vi "Find Default Node Details.vi"(6 "Node Type":string(combo)="DefaultChannelNodes", 8 "error in":errorcluster, 11 "Section Node":refnum<k20>) -> (0 "error out":errorcluster, 3 "Default Node Details":cluster{"Name":string, "TypeName":string}[](array[cluster]))   [LabVIEW 2025]
uses:
  <resource>/objmgr/DOMUserDefRef.rc
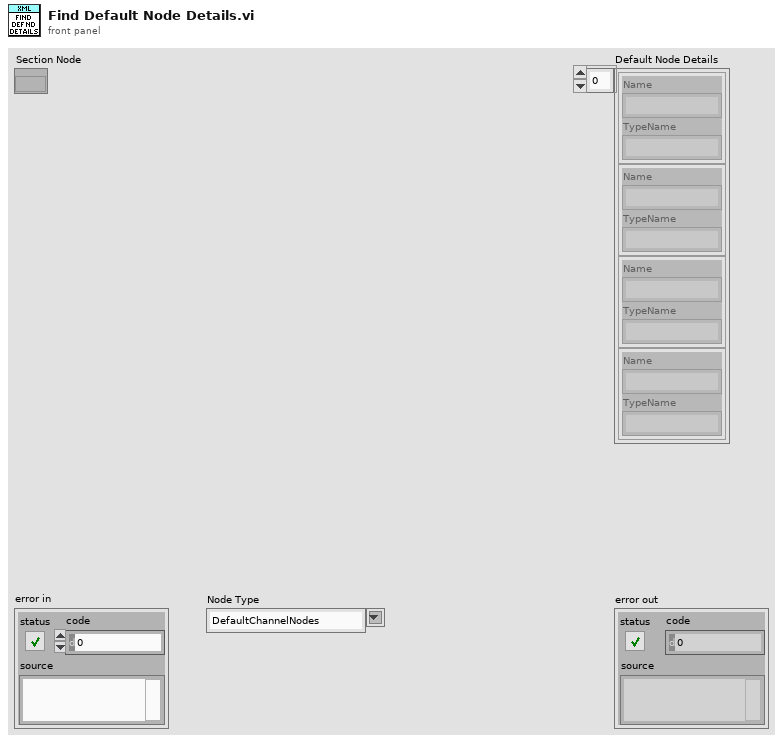
[diagram p1: front panel]
types:
  T1 = cluster{"Attribute Value":string, "Attribute Value":string}
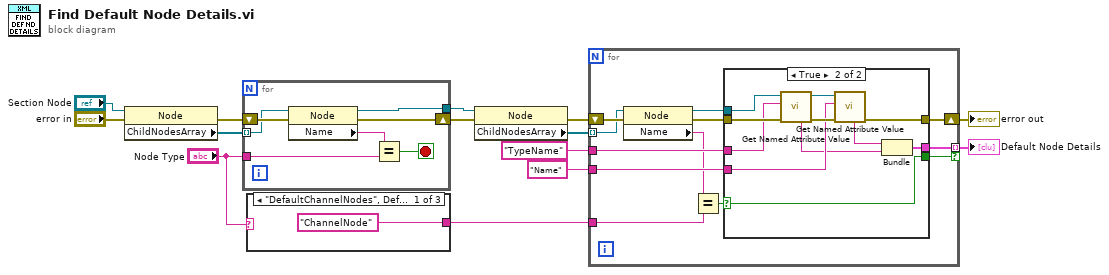
[diagram p0: block diagram]
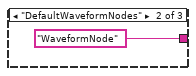
[diagram p2: hidden frame]
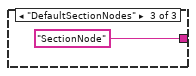
[diagram p3: hidden frame]
diagram:
  n1 = property class="Node"(reference="Section Node", error in="error in") -> (error out=w12:errorcluster, "ChildNodesArray"=w13:refnum<k20>[])  [unwired: 1 out]
  n2 = for {
    tunnel: w13 -> [w20] mode=indexing
    shift-right: [w19] -> w11
    shift-left: w12 -> [w21]
    tunnel: "Node Type" -> [w17]
    tunnel: [w15] -> w8
    stop <- w16 stop-if-true
    n3 = property class="Node"(reference=w20, error in=w21) -> (reference out=w15:refnum<k20>, error out=w19:errorcluster, "Name"=w18:string)
    n4 = Equal?(x=w18, y=w17) -> (x = y?=w16:bool)
  }
  n5 = case shown="\"DefaultChannelNodes\", Default" "Node Type" {
    tunnel: ["ChannelNode" "WaveformNode" "SectionNode"] -> w2
    frame "DefaultChannelNodes", Default {
    }
    frame "DefaultWaveformNodes" {
    }
    frame "DefaultSectionNodes" {
    }
  }
  n6 = property class="Node"(reference=w8, error in=w11) -> (error out=w9:errorcluster, "ChildNodesArray"=w10:refnum<k20>[])  [unwired: 1 out]
  n7 = for {
    tunnel: w10 -> [w35] mode=indexing
    shift-right: [w30] -> w1
    shift-left: w9 -> [w36]
    tunnel: "TypeName" ("Attribute Name") -> [w32]
    tunnel: "Name" ("Attribute Name") -> [w31]
    tunnel: [w29] -> w5 mode=indexing if=w28
    tunnel: w2 -> [w27]
    n8 = property class="Node"(reference=w35, error in=w36) -> (reference out=w34:refnum<k20>, error out=w33:errorcluster, "Name"=w26:string)
    n9 = Equal?(x=w26, y=w27) -> (x = y?=w25:bool)
    n10 = case shown="True" w25 {
      selector: w25 -> [_ w38]
      tunnel: w34 -> [_ w47]
      tunnel: w33 -> [w37 w48]
      tunnel: w32 -> [_ w46]
      tunnel: w31 -> [_ w43]
      tunnel: [w37 w42] -> w30
      tunnel: [_ w39] -> w29
      tunnel: [_ w38] -> w28
      frame False {
      }
      frame True {
        n11 = call "Get Named Attribute Value.vi"("error in"=w48, "Attribute Name"=w46, "Node In"=w47) -> ("error out"=w45:errorcluster, "Node Out"=w44:refnum<k20>, "Attribute Value"=w40:string)  [unwired: 5 in, 1 out]
        n12 = call "Get Named Attribute Value.vi"("error in"=w45, "Attribute Name"=w43, "Node In"=w44) -> ("error out"=w42:errorcluster, "Attribute Value"=w41:string)  [unwired: 5 in, 2 out]
        n13 = Bundle("Attribute Value"=w41, "Attribute Value"=w40) -> (w39:T1)  [unwired: 1 in]
      }
    }
  }
  "Default Node Details" <- w5
  "error out" <- w1
